vi "Gas_Density.vi"(1 "Pressure (mbars)":dbl=1013.25 format="%.2f", 2 "Temperature (deg C)":dbl format="%.2f", 3 "Gas Name":string) -> (0 "Density Kg/m3":dbl format="%.4f")   [LabVIEW 2010]
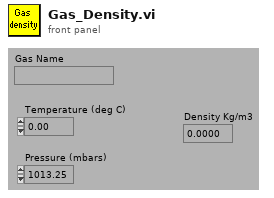
[diagram p1: front panel]
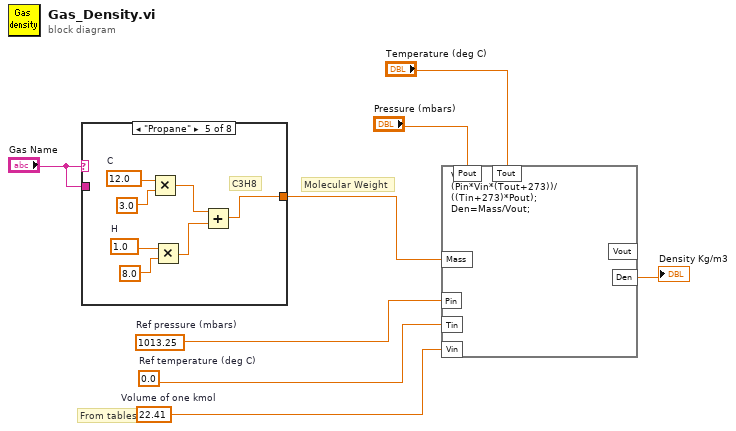
[diagram p0: block diagram]
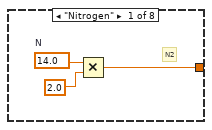
[diagram p2: hidden frame]
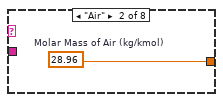
[diagram p3: hidden frame]
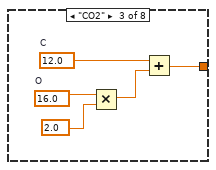
[diagram p4: hidden frame]
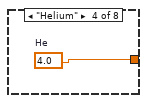
[diagram p5: hidden frame]
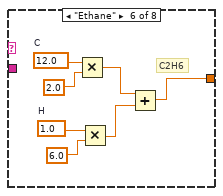
[diagram p6: hidden frame]
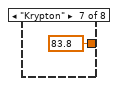
[diagram p7: hidden frame]
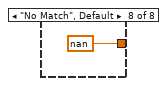
[diagram p8: hidden frame]
diagram:
  w6 = 1013.25  # Ref pressure (mbars)
  w5 = 0.0  # Ref temperature (deg C)
  w8 = 22.41  # Volume of one kmol
  # "Molecular Weight"
  # "From tables"
  n1 = case shown="\"Propane\"" "Gas Name" {
    tunnel: [w9 w12 w13 w18 w19 w26 83.8 nan] -> w7
    tunnel: "Gas Name" -> [_ _ _ _ _ _ _ _]
    frame "Nitrogen" {
      w11 = 14.0  # N
      # "N2"
      n2 = Multiply(x=w11, y=2.0) -> (x*y=w9:dbl)
    }
    frame "Air" {
      w12 = 28.96  # Molar Mass of Air (kg/kmol)
    }
    frame "CO2" {
      w17 = 12.0  # C
      w14 = 16.0  # O
      n3 = Multiply(x=w14, y=2.0 ("O")) -> (x*y=w16:dbl)
      n4 = Add(x=w17, y=w16) -> (x+y=w13:dbl)
    }
    frame "Helium" {
      w18 = 4.0  # He
    }
    frame "Propane" {
      w23 = 1.0  # H
      w24 = 12.0  # C
      # "C3H8"
      n5 = Multiply(x=w24, y=3.0) -> (x*y=w21:dbl)
      n6 = Multiply(x=w23, y=8.0) -> (x*y=w20:dbl)
      n7 = Add(x=w21, y=w20) -> (x+y=w19:dbl)
    }
    frame "Ethane" {
      w30 = 1.0  # H
      w31 = 12.0  # C
      # "C2H6"
      n8 = Multiply(x=w31, y=2.0) -> (x*y=w28:dbl)
      n9 = Multiply(x=w30, y=6.0) -> (x*y=w27:dbl)
      n10 = Add(x=w28, y=w27) -> (x+y=w26:dbl)
    }
    frame "Krypton" {
    }
    frame "No Match", Default {
    }
  }
  n11 = formula code="Vout=\n(Pin*Vin*(Tout+273))/((Tin+273)*Pout);\nDen=Mass/Vout;"("Pin"=w6, "Vin"=w8, "Tout"="Temperature (deg C)", "Tin"=w5, "Pout"="Pressure (mbars)", "Mass"=w7) -> ("Den"=→"Density Kg/m3":dbl)  [unwired: 1 out]
